vi "filter spot locations.vi"(7 "high cutoff freq: fh":dbl=0.45000000000000007 format="%0.3f", 9 "sampling freq: fs":dbl=1.0 format="%0.2f", 10 "Spot locations":T2(array[cluster])=[{"x value"=0, "y value"=0, "z value"=0}, {"x value"=0, "y value"=0, "z value"=0}, {"x value"=0, "y value"=0, "z value"=0}, {"x value"=0, "y value"=0, "z value"=0}]) -> (2 "filtered spot locations":T1(array[cluster]))   [LabVIEW 2010]
uses:
  <vilib>/ptbypt/NI_PtbyPt.lvlib
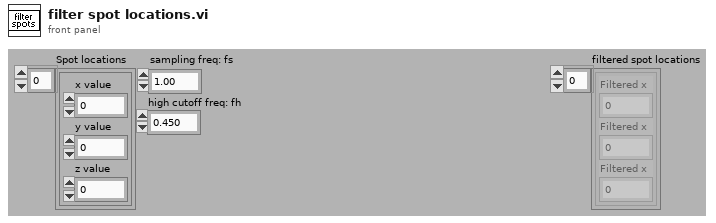
[diagram p1: front panel]
types:
  T1 = cluster{"Filtered x":dbl, "Filtered x":dbl, "Filtered x":dbl}[]
  T2 = cluster{"x value":i16, "y value":i16, "z value":i16}[]
  T3 = cluster{"Spot locations[0]":cluster{"x value":i16, "y value":i16, "z value":i16}, "Spot locations[1]":cluster{"x value":i16, "y value":i16, "z value":i16}, "Spot locations[2]":cluster{"x value":i16, "y value":i16, "z value":i16}, "Spot locations[3]":cluster{"x value":i16, "y value":i16, "z value":i16}}
  T4 = cluster{"x value":i16, "y value":i16, "z value":i16}
  T5 = cluster{"Filtered x":dbl, "Filtered x":dbl, "Filtered x":dbl}
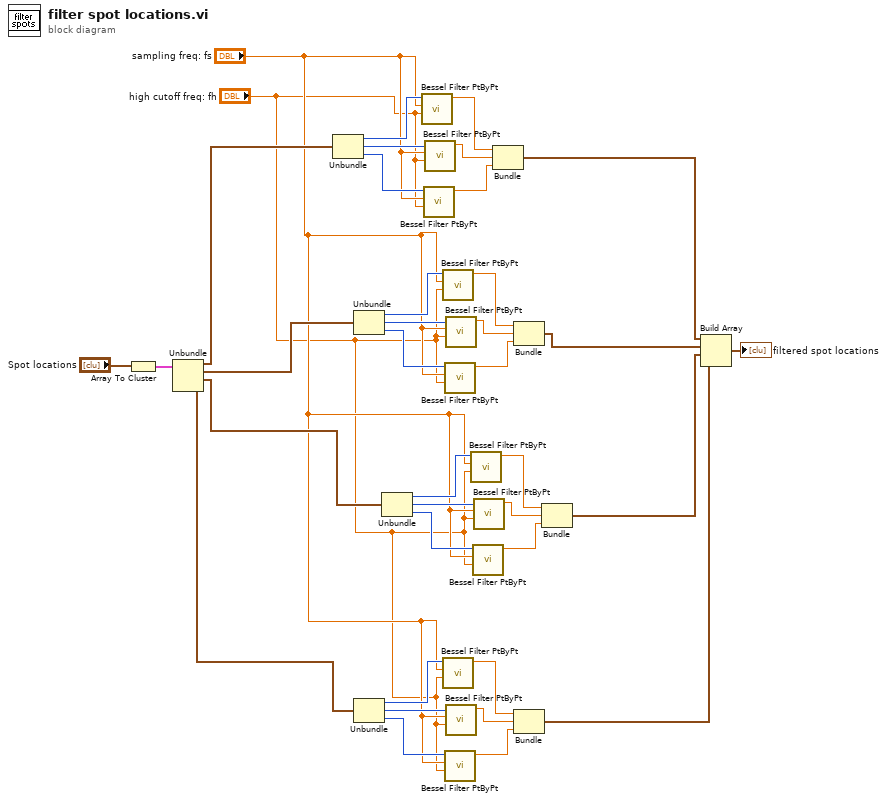
[diagram p0: block diagram]
diagram:
  n1 = Array To Cluster(array="Spot locations") -> (cluster=w36:T3)
  n2 = Unbundle(w36) -> ("Spot locations[0]"=w35:T4, "Spot locations[1]"=w22:T4, "Spot locations[2]"=w15:T4, "Spot locations[3]"=w8:T4)
  n3 = Unbundle(w35) -> ("x value"=w34:i16, "y value"=w33:i16, "z value"=w32:i16)
  n4 = Unbundle(w22) -> ("x value"=w28:i16, "y value"=w27:i16, "z value"=w26:i16)
  n5 = Unbundle(w8) -> ("x value"=w14:i16, "y value"=w13:i16, "z value"=w12:i16)
  n6 = Unbundle(w15) -> ("x value"=w21:i16, "y value"=w20:i16, "z value"=w19:i16)
  n7 = call <vilib>:"Bessel Filter PtByPt.vi"("high cutoff freq: fh"="high cutoff freq: fh", "sampling freq: fs"="sampling freq: fs", "x"=w34) -> ("Filtered x"=w31:dbl)  [unwired: 6 in, 1 out]
  n8 = call <vilib>:"Bessel Filter PtByPt.vi"("high cutoff freq: fh"="high cutoff freq: fh", "sampling freq: fs"="sampling freq: fs", "x"=w32) -> ("Filtered x"=w29:dbl)  [unwired: 6 in, 1 out]
  n9 = call <vilib>:"Bessel Filter PtByPt.vi"("high cutoff freq: fh"="high cutoff freq: fh", "sampling freq: fs"="sampling freq: fs", "x"=w33) -> ("Filtered x"=w30:dbl)  [unwired: 6 in, 1 out]
  n10 = call <vilib>:"Bessel Filter PtByPt.vi"("high cutoff freq: fh"="high cutoff freq: fh", "sampling freq: fs"="sampling freq: fs", "x"=w28) -> ("Filtered x"=w25:dbl)  [unwired: 6 in, 1 out]
  n11 = call <vilib>:"Bessel Filter PtByPt.vi"("high cutoff freq: fh"="high cutoff freq: fh", "sampling freq: fs"="sampling freq: fs", "x"=w14) -> ("Filtered x"=w11:dbl)  [unwired: 6 in, 1 out]
  n12 = call <vilib>:"Bessel Filter PtByPt.vi"("high cutoff freq: fh"="high cutoff freq: fh", "sampling freq: fs"="sampling freq: fs", "x"=w26) -> ("Filtered x"=w23:dbl)  [unwired: 6 in, 1 out]
  n13 = call <vilib>:"Bessel Filter PtByPt.vi"("high cutoff freq: fh"="high cutoff freq: fh", "sampling freq: fs"="sampling freq: fs", "x"=w12) -> ("Filtered x"=w9:dbl)  [unwired: 6 in, 1 out]
  n14 = call <vilib>:"Bessel Filter PtByPt.vi"("high cutoff freq: fh"="high cutoff freq: fh", "sampling freq: fs"="sampling freq: fs", "x"=w27) -> ("Filtered x"=w24:dbl)  [unwired: 6 in, 1 out]
  n15 = call <vilib>:"Bessel Filter PtByPt.vi"("high cutoff freq: fh"="high cutoff freq: fh", "sampling freq: fs"="sampling freq: fs", "x"=w13) -> ("Filtered x"=w10:dbl)  [unwired: 6 in, 1 out]
  n16 = call <vilib>:"Bessel Filter PtByPt.vi"("high cutoff freq: fh"="high cutoff freq: fh", "sampling freq: fs"="sampling freq: fs", "x"=w21) -> ("Filtered x"=w18:dbl)  [unwired: 6 in, 1 out]
  n17 = call <vilib>:"Bessel Filter PtByPt.vi"("high cutoff freq: fh"="high cutoff freq: fh", "sampling freq: fs"="sampling freq: fs", "x"=w19) -> ("Filtered x"=w16:dbl)  [unwired: 6 in, 1 out]
  n18 = call <vilib>:"Bessel Filter PtByPt.vi"("high cutoff freq: fh"="high cutoff freq: fh", "sampling freq: fs"="sampling freq: fs", "x"=w20) -> ("Filtered x"=w17:dbl)  [unwired: 6 in, 1 out]
  n19 = Bundle("Filtered x"=w31, "Filtered x"=w30, "Filtered x"=w29) -> (w5:T5)  [unwired: 1 in]
  n20 = Bundle("Filtered x"=w25, "Filtered x"=w24, "Filtered x"=w23) -> (w4:T5)  [unwired: 1 in]
  n21 = Bundle("Filtered x"=w11, "Filtered x"=w10, "Filtered x"=w9) -> (w2:T5)  [unwired: 1 in]
  n22 = Bundle("Filtered x"=w18, "Filtered x"=w17, "Filtered x"=w16) -> (w3:T5)  [unwired: 1 in]
  n23 = Build Array(w5, w4, w3, w2) -> (→"filtered spot locations":T1)
